vi "CreateTestTag.vi"(10 "TestCaseId":string, 11 "SuitesRunning":string[](array[string])) -> (1 "TestTagListBox":string, 2 "TestTagTree":string)   [LabVIEW 2009, in "GraphicalTestRunner.lvlib"]
uses:
  GraphicalTestRunner.lvlib
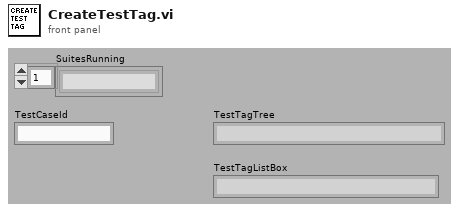
[diagram p1: front panel]
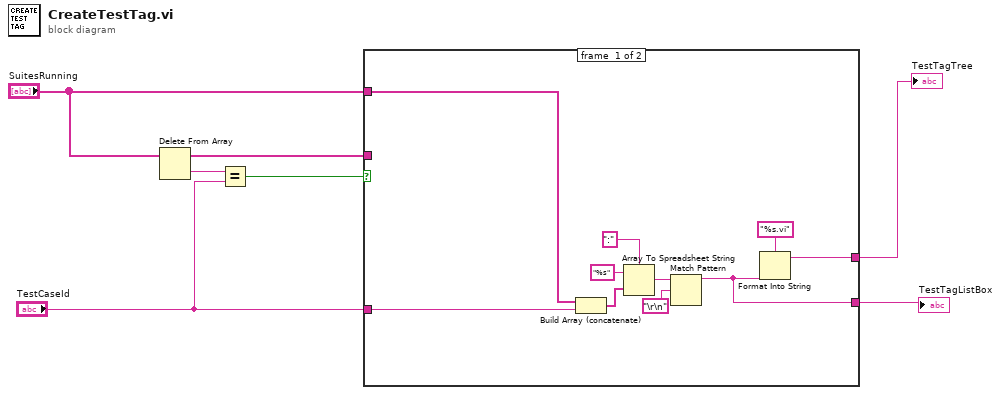
[diagram p0: block diagram]
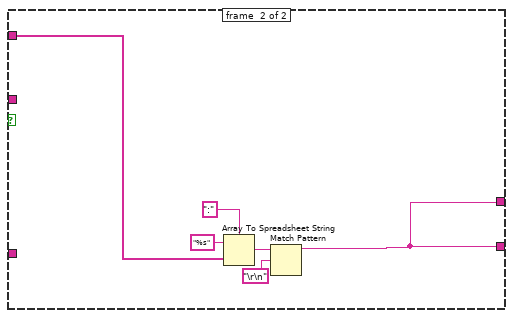
[diagram p2: hidden frame]
diagram:
  n1 = Delete From Array(array="SuitesRunning") -> (deleted portion=w4:string, array with subset deleted=w1:string[])  [unwired: 2 in]
  n2 = Equal?(x=w4, y="TestCaseId") -> (x = y?=w2:bool)
  n3 = case shown="True" w2 {
    tunnel: [w11 w18] -> w7
    tunnel: [w10 w18] -> w6
    tunnel: "SuitesRunning" -> [w9 w19]
    tunnel: "TestCaseId" -> [w8 _]
    tunnel: w1 -> [_ _]
    frame #0 {
      n4 = Build Array (concatenate)(w9, w8) -> (w17:string[])
      n5 = Array To Spreadsheet String(delimiter (Tab)=":", array=w17, 3:"%s" ("format string")) -> (spreadsheet string=w15:string)
      n6 = Match Pattern(string=w15, regular expression="\r\n") -> (before substring=w11:string)  [unwired: 1 in, 3 out]
      n7 = Format Into String(format string="%s.vi", w11) -> (resulting string=w10:string)  [unwired: 2 in, 1 out]
    }
    frame #1 {
      n8 = Array To Spreadsheet String(delimiter (Tab)=":", array=w19, 3:"%s" ("format string")) -> (spreadsheet string=w22:string)
      n9 = Match Pattern(string=w22, regular expression="\r\n") -> (before substring=w18:string)  [unwired: 1 in, 3 out]
    }
  }
  "TestTagTree" <- w6
  "TestTagListBox" <- w7
